vi "ACQ Start2.vi"(8 "error in (no error)":errorcluster, 11 "VISA resource name In":T1={"Conection Data"="COM4"}) -> (0 "error out":errorcluster, 3 "VISA resource name Out":T1={"Conection Data"="COM4"})   [LabVIEW 2014, in "AD4212C Lib.lvlib"]
doc: "Detiene la adquisición de datos, limpia la UART y reinicia la adquisición."
uses:
  AD4212C Lib.lvlib
  Typedef/Connection Data.ctl
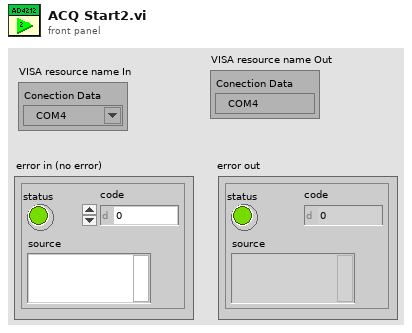
[diagram p1: front panel]
types:
  T1 = typedef "AD4212C Lib.lvlib/Connection Data.ctl" = cluster{"Conection Data":refnum<visa-resource-name>}
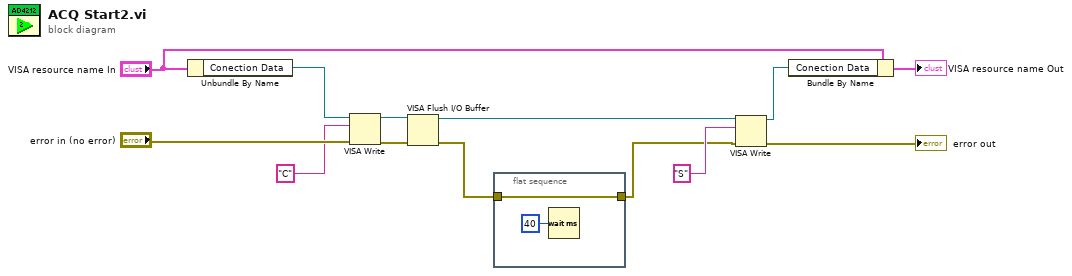
[diagram p0: block diagram]
diagram:
  n1 = Unbundle By Name("VISA resource name In") -> ("Conection Data"=w6:refnum<visa-resource-name>)
  n2 = VISA Write(VISA resource name=w6, write buffer="C", error in (no error)="error in (no error)") -> (VISA resource name out=w13:refnum<visa-resource-name>, error out=w7:errorcluster)  [unwired: 1 out]
  n3 = VISA Flush I/O Buffer(VISA resource name=w13, error in (no error)=w7) -> (VISA resource name out=w9:refnum<visa-resource-name>, error out=w2:errorcluster)  [unwired: 1 in]
  n4 = flat-sequence {
    tunnel: [w15] -> w1
    tunnel: w2 -> [w15]
    frame #0 {
      n5 = Wait (ms)(milliseconds to wait=u32 40) -> ()  [unwired: 1 out]
    }
  }
  n6 = VISA Write(VISA resource name=w9, write buffer="S", error in (no error)=w1) -> (VISA resource name out=w5:refnum<visa-resource-name>, error out=→"error out":errorcluster)  [unwired: 1 out]
  n7 = Bundle By Name(cluster="VISA resource name In", "Conection Data"=w5) -> (→"VISA resource name Out":T1)
